vi "SupportAttackerPosition_Init.vi"(0 "object in":refnum<class "SupportAttackerPosition.lvclass">, 5 "error in (no error)":errorcluster) -> (14 "object out":refnum<class "SupportAttackerPosition.lvclass">, 19 "error out":errorcluster)   [LabVIEW 2023, in "SupportAttackerPosition.lvclass"]
uses:
  SupportAttackerPosition.lvclass
  C:/Users/ebert/Documents/codes/SSL/repo/SSL_AI/NewSTP/Evaluators/Evaluator_class/Evaluator.lvclass
  Criteria/OpenAngleToGoal_class/OpenAngleToGoal.lvclass
  C:/Users/ebert/Documents/codes/SSL/repo/SSL_AI/NewSTP/Criteria/Criterion_class/Criterion.lvclass
  Criteria/PassInterception_class/PassInterception.lvclass
  Criteria/OutOfGoalieArea_class/OutOfGoalieArea.lvclass
  Criteria/PassDistance_class/PassDistance.lvclass
  Criteria/ShotInterception_class/ShotInterception.lvclass
  Evaluator_class/Evaluator.lvclass
  Criteria/ReceptionAngle_class/ReceptionAngle.lvclass
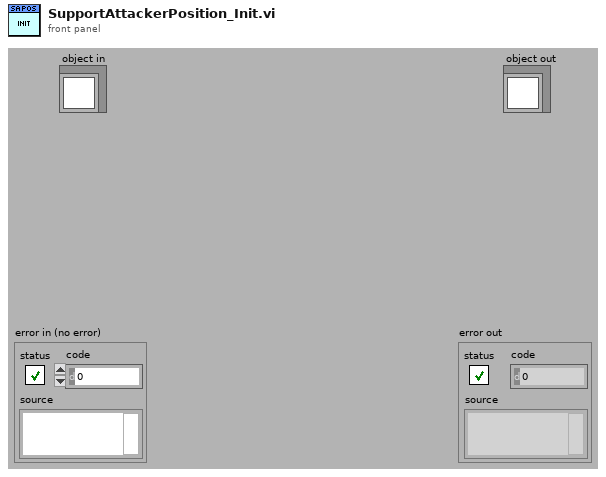
[diagram p1: front panel]
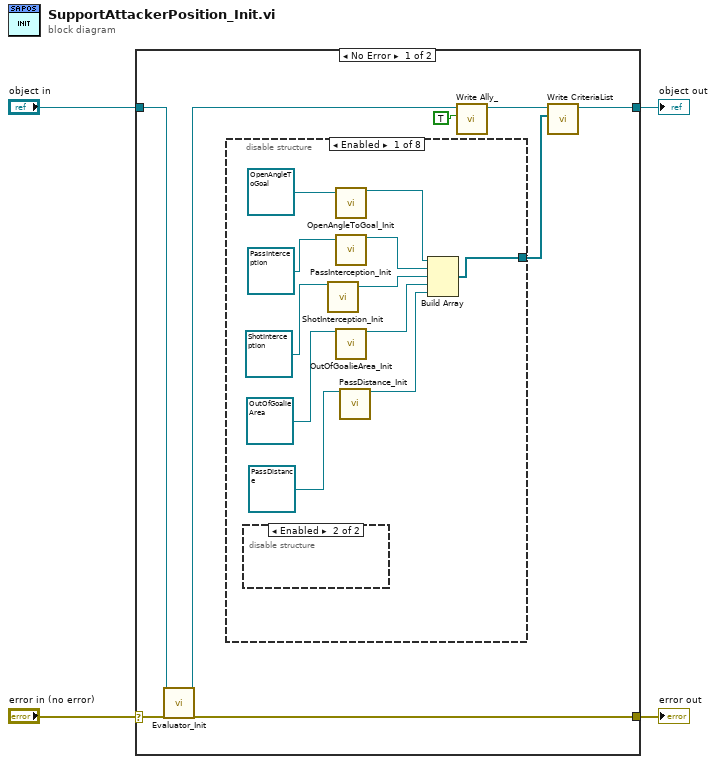
[diagram p0: block diagram]
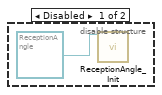
[diagram p2: hidden frame]
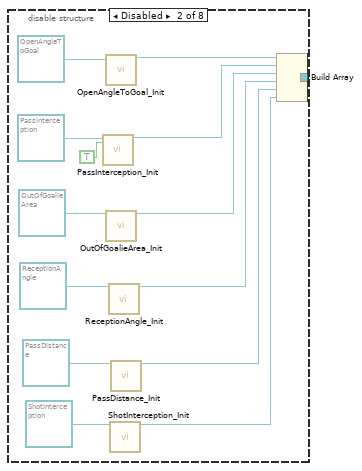
[diagram p3: hidden frame]
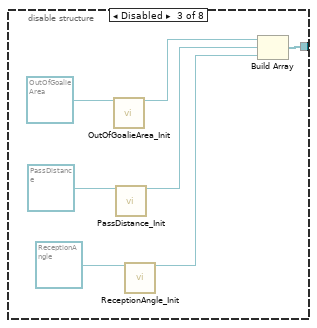
[diagram p4: hidden frame]
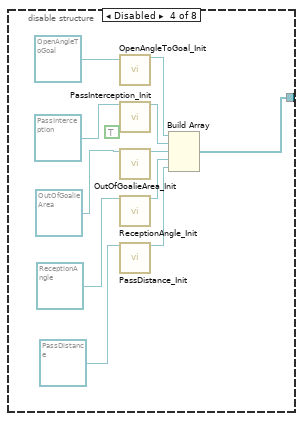
[diagram p5: hidden frame]
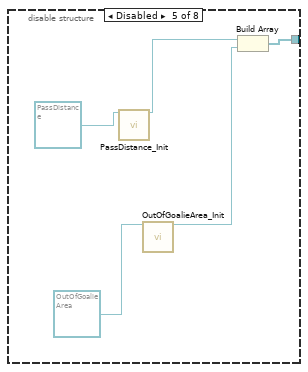
[diagram p6: hidden frame]
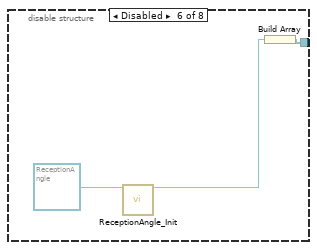
[diagram p7: hidden frame]
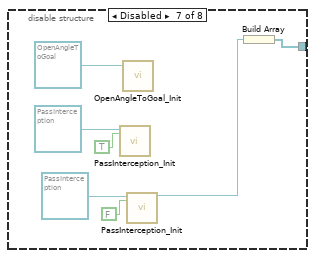
[diagram p8: hidden frame]
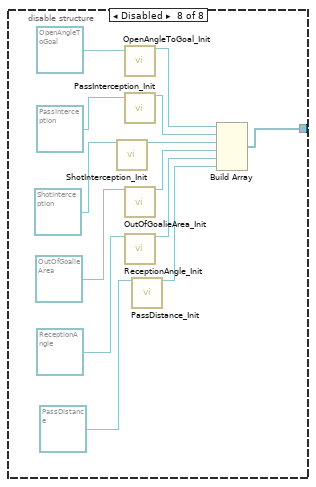
[diagram p9: hidden frame]
diagram:
  n1 = case shown="No Error" "error in (no error)" {
    selector: "error in (no error)" -> [w12 w86]
    tunnel: [w6 w87] -> w4
    tunnel: "object in" -> [w10 w87]
    tunnel: [w11 w86] -> w1
    frame No Error {
      n2 = call "Evaluator_Init.vi"("object in"=w10, "error in (no error)"=w12) -> ("object out"=w8:refnum<class "SupportAttackerPosition.lvclass">, "error out"=w11:errorcluster)  [unwired: 16 in]
      n3 = disable-structure shown="Enabled" {
        disable-tunnel: [w14 w34 w43 w51 w62 w65 w66 w75] -> w5
        frame Enabled {
          n4 = disable-structure shown="Enabled" {
            frame Disabled {
              n5 = call "ReceptionAngle_Init.vi"("object in"=refnum<class "ReceptionAngle.lvclass"> refnum ("ReceptionAngle")) -> ()  [unwired: 17 in, 2 out]
            }
            frame Enabled {
            }
          }
          n6 = call "ShotInterception_Init.vi"("object in"=refnum<class "ShotInterception.lvclass"> refnum ("ShotTime")) -> ("object out"=w16:refnum<class "ShotInterception.lvclass">)  [unwired: 17 in, 1 out]
          n7 = call "OpenAngleToGoal_Init.vi"("object in"=refnum<class "OpenAngleToGoal.lvclass"> refnum ("OpenAngleToGoal")) -> ("object out"=w18:refnum<class "OpenAngleToGoal.lvclass">)  [unwired: 17 in, 1 out]
          n8 = call "PassInterception_Init.vi"("object in"=refnum<class "PassInterception.lvclass"> refnum ("BallInterception")) -> ("object out"=w15:refnum<class "PassInterception.lvclass">)  [unwired: 17 in, 1 out]
          n9 = call "OutOfGoalieArea_Init.vi"("object in"=refnum<class "OutOfGoalieArea.lvclass"> refnum ("OutOfGoalieArea")) -> ("object out"=w17:refnum<class "OutOfGoalieArea.lvclass">)  [unwired: 17 in, 1 out]
          n10 = call "PassDistance_Init.vi"("object in"=refnum<class "PassDistance.lvclass"> refnum ("PassDistance")) -> ("object out"=w13:refnum<class "PassDistance.lvclass">)  [unwired: 17 in, 1 out]
          n11 = Build Array(w18, w15, w16, w17, w13) -> (w14:refnum<class "Criterion.lvclass">[])
        }
        frame Disabled {
          n12 = call "PassInterception_Init.vi"("object in"=refnum<class "PassInterception.lvclass"> refnum ("BallInterception"), 1:TRUE ("Pass?")) -> ("object out"=w35:refnum<class "PassInterception.lvclass">)  [unwired: 16 in, 1 out]
          n13 = call "OpenAngleToGoal_Init.vi"("object in"=refnum<class "OpenAngleToGoal.lvclass"> refnum ("OpenAngleToGoal")) -> ("object out"=w36:refnum<class "OpenAngleToGoal.lvclass">)  [unwired: 17 in, 1 out]
          n14 = call "OutOfGoalieArea_Init.vi"("object in"=refnum<class "OutOfGoalieArea.lvclass"> refnum ("OutOfGoalieArea")) -> ("object out"=w32:refnum<class "OutOfGoalieArea.lvclass">)  [unwired: 17 in, 1 out]
          n15 = call "ReceptionAngle_Init.vi"("object in"=refnum<class "ReceptionAngle.lvclass"> refnum ("ReceptionAngle")) -> ("object out"=w30:refnum<class "ReceptionAngle.lvclass">)  [unwired: 17 in, 1 out]
          n16 = call "ShotInterception_Init.vi"("object in"=refnum<class "ShotInterception.lvclass"> refnum ("ShotTime")) -> ("object out"=w26:refnum<class "ShotInterception.lvclass">)  [unwired: 17 in, 1 out]
          n17 = call "PassDistance_Init.vi"("object in"=refnum<class "PassDistance.lvclass"> refnum ("PassDistance")) -> ("object out"=w28:refnum<class "PassDistance.lvclass">)  [unwired: 17 in, 1 out]
          n18 = Build Array(w36, w35, w32, w30, w28, w26) -> (w34:refnum<class "Criterion.lvclass">[])
        }
        frame Disabled {
          n19 = call "OutOfGoalieArea_Init.vi"("object in"=refnum<class "OutOfGoalieArea.lvclass"> refnum ("OutOfGoalieArea")) -> ("object out"=w44:refnum<class "OutOfGoalieArea.lvclass">)  [unwired: 17 in, 1 out]
          n20 = call "PassDistance_Init.vi"("object in"=refnum<class "PassDistance.lvclass"> refnum ("PassDistance")) -> ("object out"=w41:refnum<class "PassDistance.lvclass">)  [unwired: 17 in, 1 out]
          n21 = call "ReceptionAngle_Init.vi"("object in"=refnum<class "ReceptionAngle.lvclass"> refnum ("ReceptionAngle")) -> ("object out"=w39:refnum<class "ReceptionAngle.lvclass">)  [unwired: 17 in, 1 out]
          n22 = Build Array(w44, w41, w39) -> (w43:refnum<class "Criterion.lvclass">[])
        }
        frame Disabled {
          n23 = call "OpenAngleToGoal_Init.vi"("object in"=refnum<class "OpenAngleToGoal.lvclass"> refnum ("OpenAngleToGoal")) -> ("object out"=w50:refnum<class "OpenAngleToGoal.lvclass">)  [unwired: 17 in, 1 out]
          n24 = call "PassInterception_Init.vi"("object in"=refnum<class "PassInterception.lvclass"> refnum ("BallInterception"), 1:TRUE ("Pass?")) -> ("object out"=w49:refnum<class "PassInterception.lvclass">)  [unwired: 16 in, 1 out]
          n25 = call "OutOfGoalieArea_Init.vi"("object in"=refnum<class "OutOfGoalieArea.lvclass"> refnum ("OutOfGoalieArea")) -> ("object out"=w48:refnum<class "OutOfGoalieArea.lvclass">)  [unwired: 17 in, 1 out]
          n26 = call "ReceptionAngle_Init.vi"("object in"=refnum<class "ReceptionAngle.lvclass"> refnum ("ReceptionAngle")) -> ("object out"=w47:refnum<class "ReceptionAngle.lvclass">)  [unwired: 17 in, 1 out]
          n27 = call "PassDistance_Init.vi"("object in"=refnum<class "PassDistance.lvclass"> refnum ("PassDistance")) -> ("object out"=w46:refnum<class "PassDistance.lvclass">)  [unwired: 17 in, 1 out]
          n28 = Build Array(w50, w49, w48, w47, w46) -> (w51:refnum<class "Criterion.lvclass">[])
        }
        frame Disabled {
          n29 = call "PassDistance_Init.vi"("object in"=refnum<class "PassDistance.lvclass"> refnum ("PassDistance")) -> ("object out"=w60:refnum<class "PassDistance.lvclass">)  [unwired: 17 in, 1 out]
          n30 = call "OutOfGoalieArea_Init.vi"("object in"=refnum<class "OutOfGoalieArea.lvclass"> refnum ("OutOfGoalieArea")) -> ("object out"=w58:refnum<class "OutOfGoalieArea.lvclass">)  [unwired: 17 in, 1 out]
          n31 = Build Array(w60, w58) -> (w62:refnum<class "Criterion.lvclass">[])
        }
        frame Disabled {
          n32 = call "ReceptionAngle_Init.vi"("object in"=refnum<class "ReceptionAngle.lvclass"> refnum ("ReceptionAngle")) -> ("object out"=w63:refnum<class "ReceptionAngle.lvclass">)  [unwired: 17 in, 1 out]
          n33 = Build Array(w63) -> (w65:refnum<class "ReceptionAngle.lvclass">[])
        }
        frame Disabled {
          n34 = call "PassInterception_Init.vi"("object in"=refnum<class "PassInterception.lvclass"> refnum ("BallInterception"), 1:TRUE ("Pass?")) -> ()  [unwired: 16 in, 2 out]
          n35 = call "OpenAngleToGoal_Init.vi"("object in"=refnum<class "OpenAngleToGoal.lvclass"> refnum ("OpenAngleToGoal")) -> ()  [unwired: 17 in, 2 out]
          n36 = call "PassInterception_Init.vi"("object in"=refnum<class "PassInterception.lvclass"> refnum ("BallInterception"), 1:FALSE ("Pass?")) -> ("object out"=w67:refnum<class "PassInterception.lvclass">)  [unwired: 16 in, 1 out]
          n37 = Build Array(w67) -> (w66:refnum<class "PassInterception.lvclass">[])
        }
        frame Disabled {
          n38 = call "ShotInterception_Init.vi"("object in"=refnum<class "ShotInterception.lvclass"> refnum ("ShotTime")) -> ("object out"=w73:refnum<class "ShotInterception.lvclass">)  [unwired: 17 in, 1 out]
          n39 = call "OpenAngleToGoal_Init.vi"("object in"=refnum<class "OpenAngleToGoal.lvclass"> refnum ("OpenAngleToGoal")) -> ("object out"=w80:refnum<class "OpenAngleToGoal.lvclass">)  [unwired: 17 in, 1 out]
          n40 = call "PassInterception_Init.vi"("object in"=refnum<class "PassInterception.lvclass"> refnum ("BallInterception")) -> ("object out"=w79:refnum<class "PassInterception.lvclass">)  [unwired: 17 in, 1 out]
          n41 = call "OutOfGoalieArea_Init.vi"("object in"=refnum<class "OutOfGoalieArea.lvclass"> refnum ("OutOfGoalieArea")) -> ("object out"=w78:refnum<class "OutOfGoalieArea.lvclass">)  [unwired: 17 in, 1 out]
          n42 = call "ReceptionAngle_Init.vi"("object in"=refnum<class "ReceptionAngle.lvclass"> refnum ("ReceptionAngle")) -> ("object out"=w77:refnum<class "ReceptionAngle.lvclass">)  [unwired: 17 in, 1 out]
          n43 = call "PassDistance_Init.vi"("object in"=refnum<class "PassDistance.lvclass"> refnum ("PassDistance")) -> ("object out"=w76:refnum<class "PassDistance.lvclass">)  [unwired: 17 in, 1 out]
          n44 = Build Array(w80, w79, w73, w78, w77, w76) -> (w75:refnum<class "Criterion.lvclass">[])
        }
      }
      n45 = call-dynamic "Write Ally_.vi"("Ally?"=TRUE, "Evaluator in"=w8) -> ("Evaluator out"=w7:refnum<class "SupportAttackerPosition.lvclass">)  [unwired: 8 in, 1 out]
      n46 = call-dynamic "Write CriteriaList.vi"("CriteriaList"=w5, "Evaluator in"=w7) -> ("Evaluator out"=w6:refnum<class "SupportAttackerPosition.lvclass">)  [unwired: 8 in, 1 out]
    }
    frame Error {
    }
  }
  "object out" <- w4
  "error out" <- w1
